vi "Get Continuous Query.vi"(0 "InfluxDB in":refnum<class "Client.lvclass">, 11 "error in (no error)":errorcluster) -> (4 "InfluxDB out":refnum<class "Client.lvclass">, 6 "Results Out":refnum<class "Results.lvclass">, 15 "error out":errorcluster)   [LabVIEW 2018, in "InfluxDB Client.lvlib" / "Client.lvclass"]
doc: "Creates a database."
uses:
  Client.lvclass
  Results/Results.lvclass
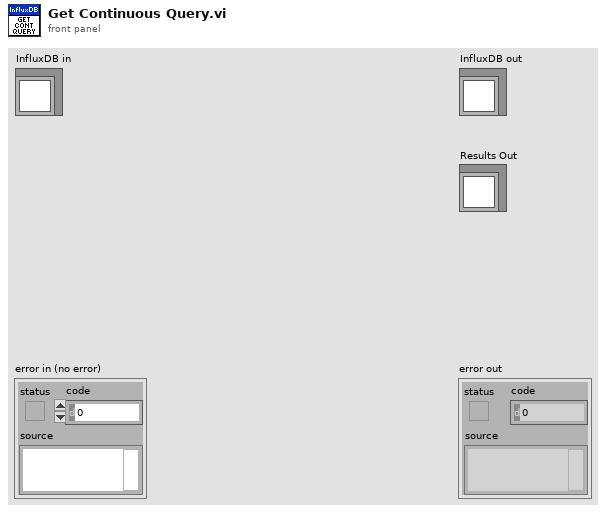
[diagram p1: front panel]
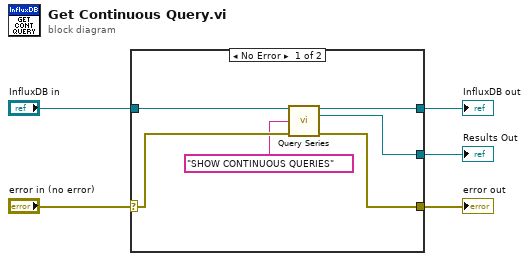
[diagram p0: block diagram]
diagram:
  n1 = case shown="No Error" "error in (no error)" {
    selector: "error in (no error)" -> [w9 w13]
    tunnel: [w6 w13] -> w4
    tunnel: [w10 w12] -> w2
    tunnel: "InfluxDB in" -> [w11 w12]
    tunnel: [w7 _] -> w1
    frame No Error {
      n2 = call "Query Series.vi"("InfluxDB in"=w11, "Measurement query"="SHOW CONTINUOUS QUERIES", "error in (no error)"=w9) -> ("InfluxDB out"=w10:refnum<class "Client.lvclass">, "Results Out"=w7:refnum<class "Results.lvclass">, "error out"=w6:errorcluster)  [unwired: 10 in]
    }
    frame Error {
    }
  }
  "error out" <- w4
  "InfluxDB out" <- w2
  "Results Out" <- w1
